vi "uninitialize.vi"(7 "ignore initialize status (T)":bool, 8 "error in (no error)":errorcluster, 11 "channel handle (0:all)":u16 format="%x") -> (0 "error out":errorcluster)   [LabVIEW 2024, in "atsj peakcan basic.lvlib"]
doc: "Uninitializes a PCAN bus (channel).\n\nCopyright (c) 2025 ATSJ (www.atsj.eu)"
uses:
  atsj peakcan basic.lvlib
  support/x64/PCANBasic.dll
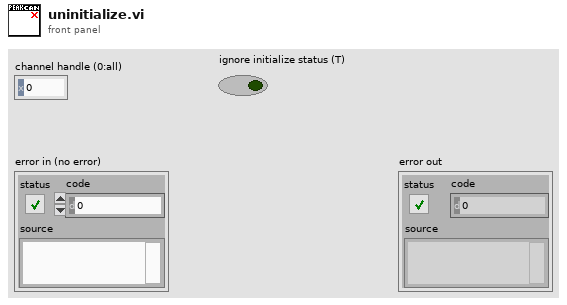
[diagram p1: front panel]
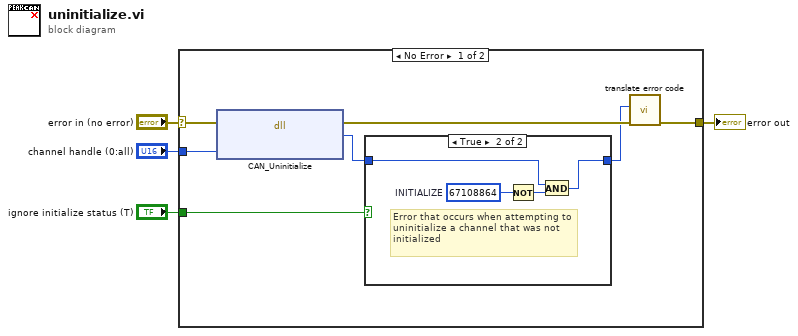
[diagram p0: block diagram]
diagram:
  n1 = case shown="No Error" "error in (no error)" {
    selector: "error in (no error)" -> [w10 w17]
    tunnel: [w6 w17] -> w3
    tunnel: "channel handle (0:all)" -> [w11 _]
    tunnel: "ignore initialize status (T)" -> [w5 _]
    frame No Error {
      n2 = dll-call lib="C:/atsj/plateau/atsj-peakcan-basic-for-labview/src/support/x64/PCANBasic.dll" fn="CAN_Uninitialize"(error in=w10, "Channel"=w11) -> (error out=w9:errorcluster, "Status"=w8:u32)  [unwired: 3 in, 1 out]
      n3 = case shown="True" w5 {
        tunnel: w8 -> [w12 w14]
        tunnel: [w12 w13] -> w7
        frame False {
        }
        frame True {
          w15 = u32 67108864  # INITIALIZE
          # "Error that occurs when attempting to uninitialize a channel that was not initialized"
          n4 = Not(x=w15) -> (.not. x?=w16:u32)
          n5 = And(x=w14, y=w16) -> (x .and. y?=w13:u32)
        }
      }
      n6 = call "translate error code.vi"("error in (no error)"=w9, "error code"=w7) -> ("error out"=w6:errorcluster)  [unwired: 9 in]
    }
    frame Error {
    }
  }
  "error out" <- w3
